vi "PidHmi.vi"() -> ()   [LabVIEW 2018]
uses:
  <vilib>/Platform/TimedLoop/XDataNode/timing_clust.ctl
  <vilib>/Platform/TimedLoop/XDataNode/nitl_modes.ctl
  <vilib>/Platform/TimedLoop/XDataNode/wakeup.ctl
  <vilib>/platform/TimedLoop/XDataNode/XDataNode.xnode
  <vilib>/Platform/TimedLoop/XDataNode/XDNodeRunTimeDep.lvlib
  ModbusTest/ModbusTestMasterHmi.lvlib
  SubVi/SubVi.lvlib
panel:
  out "error out":errorcluster
  out "Waveform Chart":dbl[][](graph)
  out "Setpoint":sgl(knob) scale=0.0..300.0
  out "Manual":i16(knob) scale=0.0..255.0
  out "Output":i16(knob) scale=0.0..255.0
  out "Temperature":sgl(slide) scale=0.0..300.0
  in  "?":T1(tab)
  out "Communication Failure":bool
  out "Off Hook":bool
  out "Updating":bool
  in  "Frequency":dbl(slide) scale=1.0..100.0
  in  "Stop":bool
  out "Counter":i32
  out "Interval":i64
  in  "file path (use dialog)":path
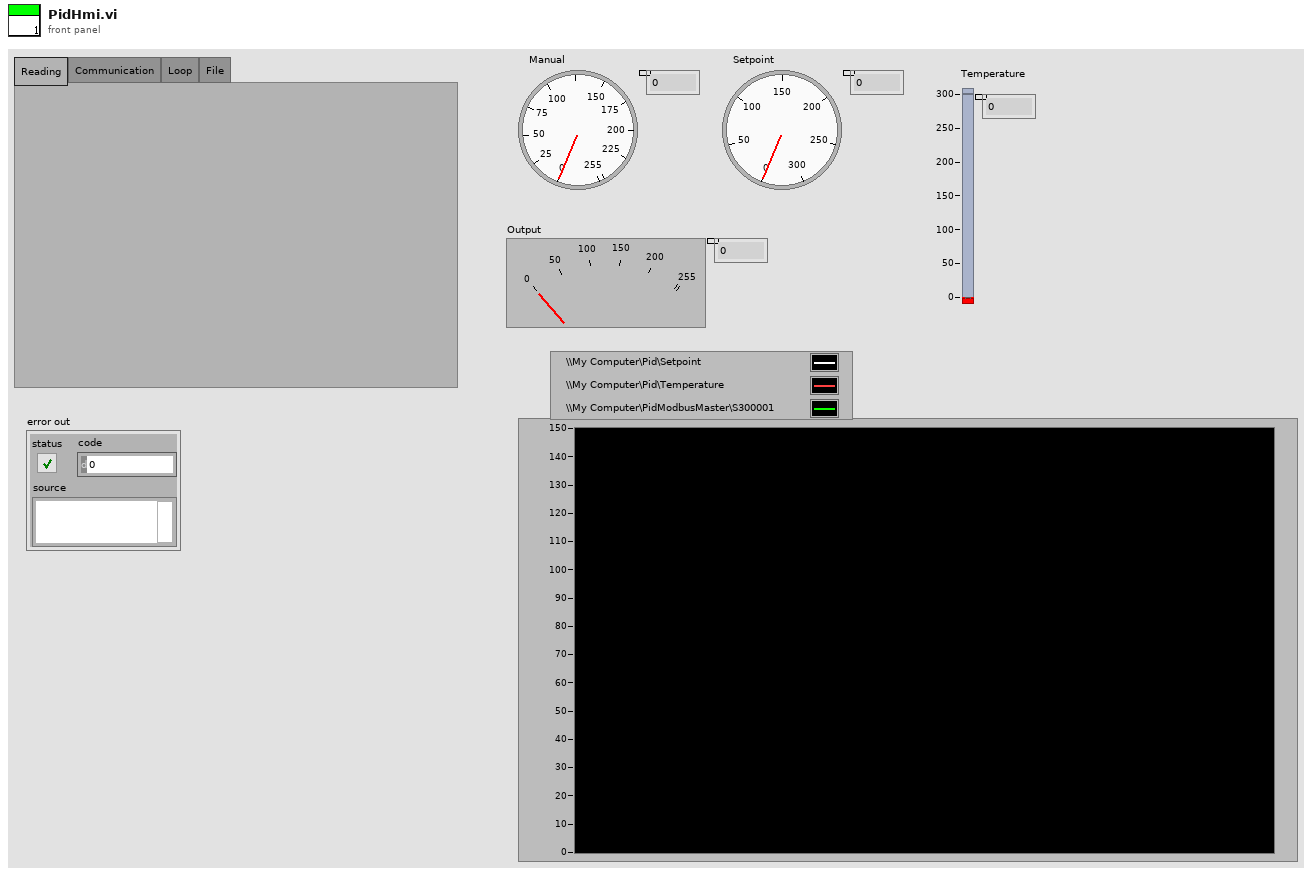
[diagram p1: front panel]
types:
  T1 = enum32{"Reading", "Communication", "Loop", "File"}
  T2 = enum16{"open", "replace", "create", "open or create", "replace or create", "replace or create with confirmation"}
  T3 = typedef "XDNodeRunTimeDep.lvlib/timing_clust.ctl" = cluster{"Expected End [f-1]":u64, "Actual End [f-1]":u64, "Finished Late? [f-1]":bool, "Expected End [i-1]":u64, "Actual End [i-1]":u64, "Finished Late? [i-1]":bool, "Expected Start [i]":u64, "Actual Start [i]":u64, "Expected Start [f]":u64, "Actual Start [f]":u64, "Source Name":string, "Structure Name":string, "Period":i64, "Deadline":i64, "Offset":i64, "Start":i64, "Priority":i32, "Timeout":i32, "Mode":T4, "Wakeup Reason":T5, "Error":errorcluster, "Source Type":string, "Secondary Source Type":string, "Global End Time":u64, "Global Start Time":u64, "Frame Duration":u64, "Iteration Duration":u64, "Assigned CPU":i32, "I/O Scan Engine Mode":u32}
  T4 = typedef "XDNodeRunTimeDep.lvlib/nitl_modes.ctl" = enum32{"No Change", "Process missed periods, maintain original phase", "Discard missed periods, maintain original phase", "Process missed periods, ignore original phase", "Discard missed periods, ignore original phase"}
  T5 = typedef "XDNodeRunTimeDep.lvlib/wakeup.ctl" = enum32{"Normal", "Aborted", "Asynchronous wakeup", "Timing source error", "Timed loop error", "Timeout"}
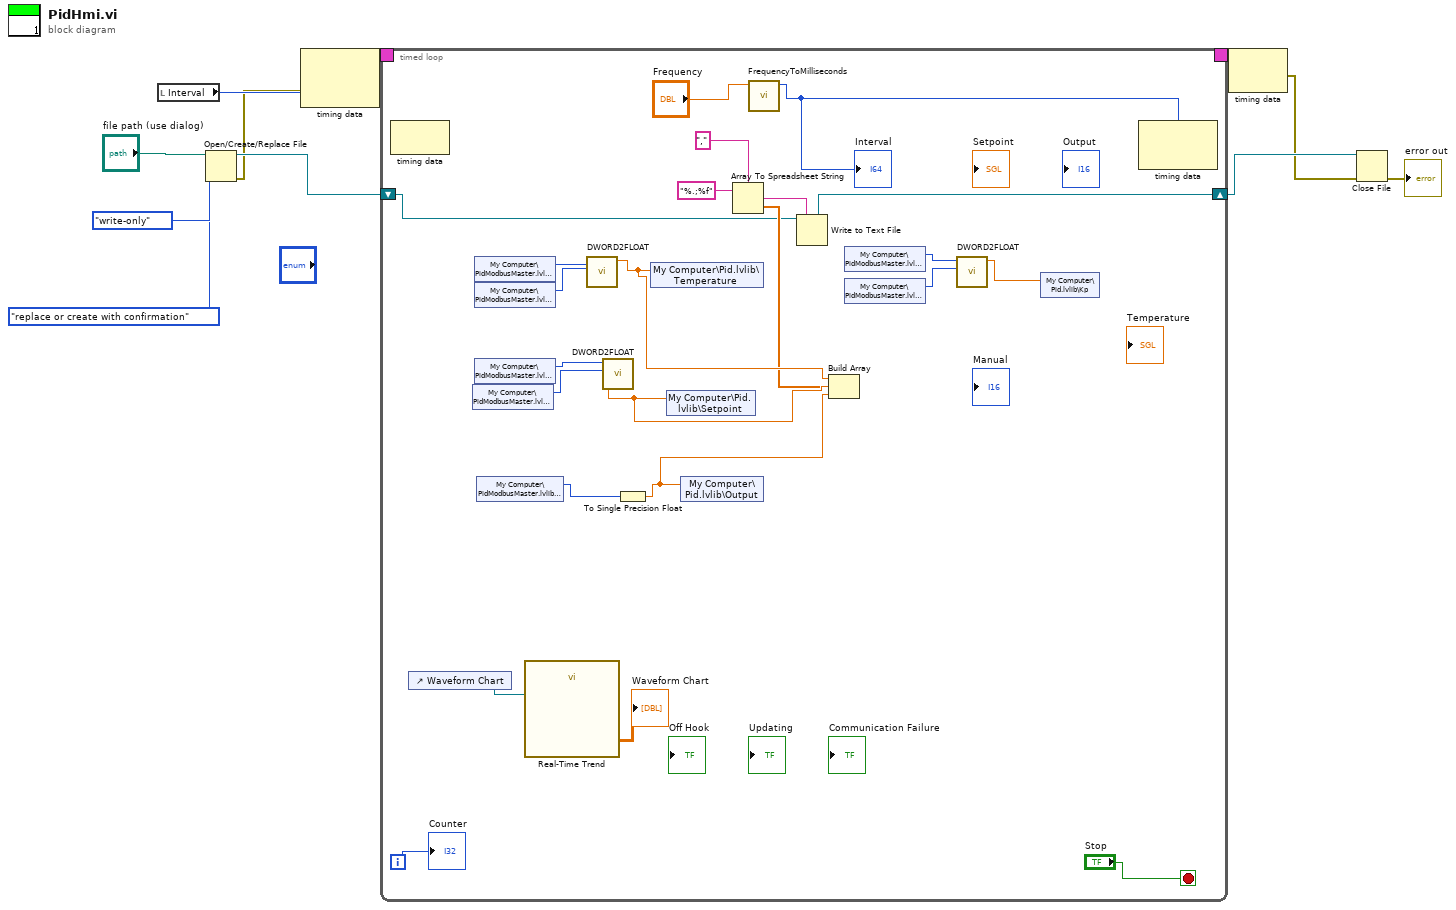
[diagram p0: block diagram]
diagram:
  n1 = local read "Interval"() -> (w9:i64)
  n2 = Open/Create/Replace File(file path (use dialog)="file path (use dialog)", operation (0:open)=T2."replace or create with confirmation", access (0:read/write)=enum16{"read/write", "read-only", "write-only"}."write-only") -> (refnum out=w8:refnum<file>, error out=w7:errorcluster)  [unwired: 3 in, 1 out]
  n3 = node-c288(w9, w7) -> (w11:T3)
  n4 = timed-loop {
    timing: w11 -> [_]
    timing-out: [_] -> w10
    shift-right: [w13] -> w3
    shift-left: w8 -> [w14]
    i -> [w34]
    stop <- "Stop" stop-if-true
    n5 = node-c288() -> ()  [unwired: 1 in, 1 out]
    n6 = control-ref of="Waveform Chart"() -> (w22:refnum<vi>)
    n7 = shared-variable "My Computer\\PidModbusMaster.lvlib\\400002"() -> (w27:u16)  [unwired: 1 in, 1 out]
    n8 = shared-variable "My Computer\\PidModbusMaster.lvlib\\300003"() -> (w30:u16)  [unwired: 1 in, 1 out]
    n9 = shared-variable "My Computer\\PidModbusMaster.lvlib\\300002"() -> (w29:u16)  [unwired: 1 in, 1 out]
    n10 = shared-variable "My Computer\\PidModbusMaster.lvlib\\400003"() -> (w28:u16)  [unwired: 1 in, 1 out]
    n11 = shared-variable "My Computer\\PidModbusMaster.lvlib\\S300001"() -> (w21:i16)  [unwired: 1 in, 1 out]
    n12 = call "Real-Time Trend"("Trend Reference"=w22) -> ("Trend Data"=→"Waveform Chart":dbl[][])  [unwired: 3 in, 7 out]
    n13 = call "DWORD2FLOAT.vi"("Low"=w29, "High"=w30) -> ("Float"=w18:sgl)  [unwired: 9 in]
    n14 = call "DWORD2FLOAT.vi"("Low"=w27, "High"=w28) -> ("Float"=w17:sgl)  [unwired: 9 in]
    n15 = To Single Precision Float(number=w21) -> (single precision float=w16:sgl)
    n16 = shared-variable "My Computer\\Pid.lvlib\\Temperature"(w18) -> ()  [unwired: 1 in, 1 out]
    n17 = shared-variable "My Computer\\Pid.lvlib\\Setpoint"(w17) -> ()  [unwired: 1 in, 1 out]
    n18 = shared-variable "My Computer\\Pid.lvlib\\Output"(w16) -> ()  [unwired: 1 in, 1 out]
    n19 = call "FrequencyToMilliseconds.vi"("Frequency"="Frequency") -> ("Numeric"=w31:i64)  [unwired: 10 in]
    "Interval" <- w31
    n20 = Build Array(w18, w17, w16) -> (w15:sgl[])
    n21 = Array To Spreadsheet String(delimiter (Tab)=",", array=w15, 3:"%.;%f" ("format string")) -> (spreadsheet string=w12:string)
    n22 = Write to Text File(file (use dialog)=w14, text=w12) -> (refnum out=w13:refnum<file>)  [unwired: 2 in, 2 out]
    n23 = shared-variable "My Computer\\PidModbusMaster.lvlib\\400005"() -> (w26:u16)  [unwired: 1 in, 1 out]
    n24 = shared-variable "My Computer\\PidModbusMaster.lvlib\\400004"() -> (w25:u16)  [unwired: 1 in, 1 out]
    n25 = call "DWORD2FLOAT.vi"("Low"=w25, "High"=w26) -> ("Float"=w24:sgl)  [unwired: 9 in]
    n26 = shared-variable "My Computer\\Pid.lvlib\\Kp"(w24) -> ()  [unwired: 1 in, 1 out]
    n27 = node-c288(w31) -> ()  [unwired: 1 in, 1 out]
    "Counter" <- w34
  }
  n28 = node-c288(w10) -> (w2:errorcluster)
  n29 = Close File(refnum=w3, error in=w2) -> (error out=→"error out":errorcluster)  [unwired: 1 out]
